vi "random numbers.vi"() -> ()   [LabVIEW 2020]
panel:
  out "random number":dbl
  in  "range":dbl
  out "number (0 to 1)":dbl
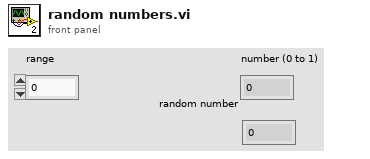
[diagram p1: front panel]
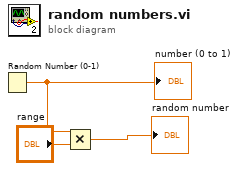
[diagram p0: block diagram]
diagram:
  n1 = Random Number (0-1)() -> (number: 0 to 1=w3:dbl)
  "number (0 to 1)" <- w3
  n2 = Multiply(x=w3, y="range") -> (x*y=→"random number":dbl)
